vi "SetN.vi"(8 "error in (no error)":errorcluster, 10 "Property":dbl, 11 "object in":refnum<class "Object (subject).lvclass">) -> (0 "error out":errorcluster, 3 "object out":refnum<class "Object (subject).lvclass">)   [LabVIEW 2014, in "Object (subject).lvclass"]
uses:
  Object (subject).lvclass
  Object (subject).lvclass/Object (subject).ctl
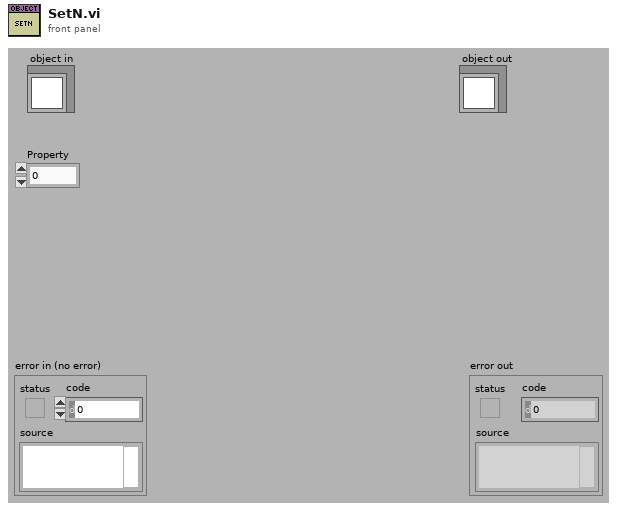
[diagram p1: front panel]
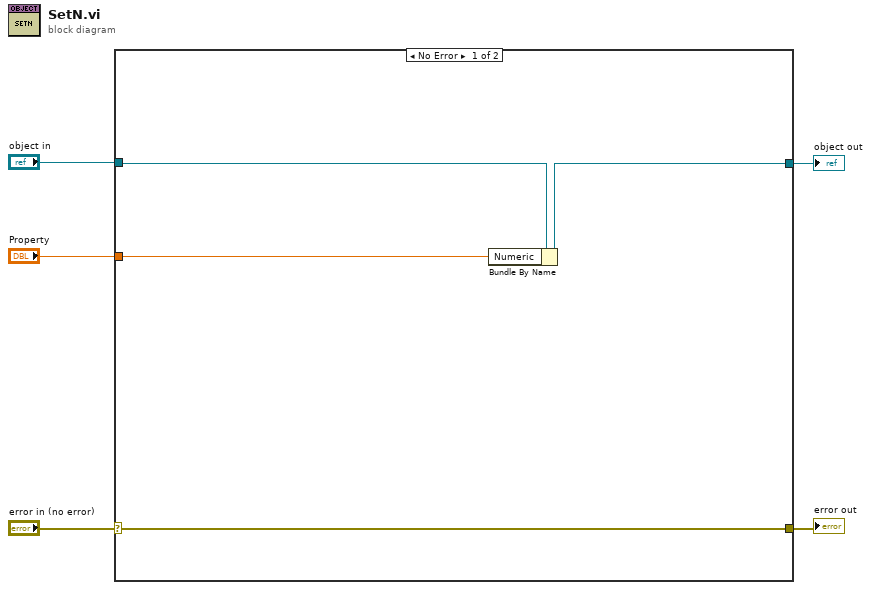
[diagram p0: block diagram]
diagram:
  n1 = case shown="No Error" "error in (no error)" {
    selector: "error in (no error)" -> [w9 w11]
    tunnel: [w9 w11] -> w4
    tunnel: [w7 w10] -> w2
    tunnel: "object in" -> [w8 w10]
    tunnel: "Property" -> [w6 _]
    frame No Error {
      n2 = Bundle By Name(cluster=w8, "Numeric"=w6) -> (w7:refnum<class "Object (subject).lvclass">)
    }
    frame Error {
    }
  }
  "error out" <- w4
  "object out" <- w2
